vi "Config_Populate.vi"(8 "error in (no error)":errorcluster, 11 "Config Ref In":T1) -> (0 "error out":errorcluster, 3 "refnum out":T1)   [LabVIEW 2021]
uses:
  <vilib>/Utility/config.llb/Config Data RefNum.ctl
  Config_Cluster.ctl
  Mode_Enum.ctl
  <vilib>/Utility/config.llb/Write Key (Path).vi
  <vilib>/Utility/config.llb/Write Key (String).vi
  <vilib>/Utility/config.llb/NI_LVConfig.lvlib
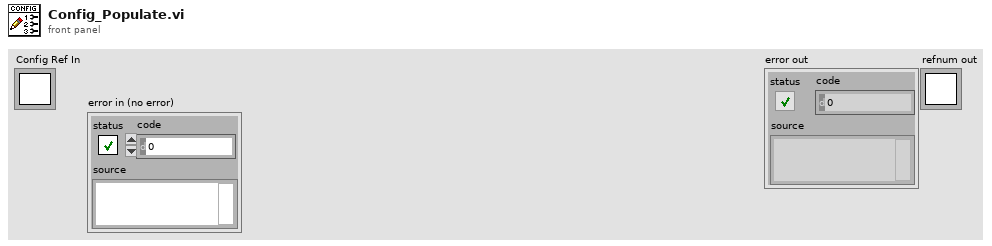
[diagram p1: front panel]
types:
  T1 = typedef "NI_LVConfig.lvlib/Config Data RefNum.ctl" = refnum<k1>
  T2 = typedef "Config_Cluster.ctl" = cluster{"General":cluster{"Config.ini":path, "Default Logging Path":path}, "Hardware":cluster{"Global T VAR":refnum<k21>, "Global B VAR":refnum<k21>, "VISAS":cluster{"GEN COM":refnum<visa-resource-name>, "SCOPE COM":refnum<visa-resource-name>, "VNA COM":refnum<visa-resource-name>}}, "Operation":cluster{"Operation Mode":T3, "Status":string, "NewLog?":bool, "OvenWarn":bool, "Scope Settings":cluster{"TimeBase":dbl, "VerticalScale":dbl}}}
  T3 = typedef "Mode_Enum.ctl" = enum16{"OvenNRDY", "Logging", "Idle-Off", "Idle"}
  T4 = cluster{"Config.ini":path, "Default Logging Path":path}
  T5 = cluster{"Global T VAR":refnum<k21>, "Global B VAR":refnum<k21>, "VISAS":cluster{"GEN COM":refnum<visa-resource-name>, "SCOPE COM":refnum<visa-resource-name>, "VNA COM":refnum<visa-resource-name>}}
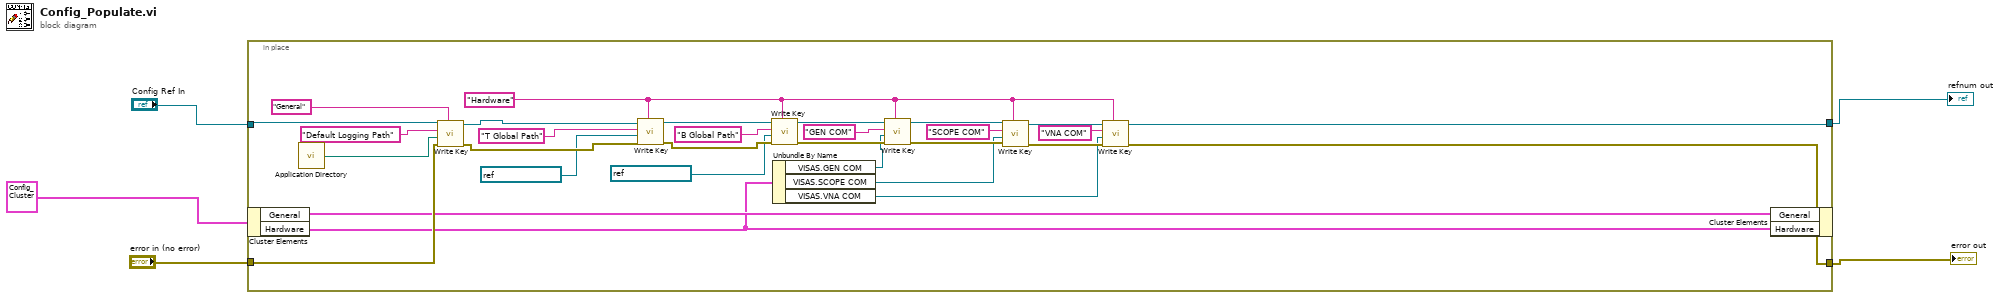
[diagram p0: block diagram]
diagram:
  n1 = in-place {
    in-place-border: "Config Ref In" -> [w35]
    in-place-border: "error in (no error)" -> [w34]
    in-place-border: [w7] -> w2
    in-place-border: [w6] -> w1
    w8 = "Hardware" ("section")
    n2 = in-place-cluster #1(T2 {"General"={"Config.ini"=path "", "Default Logging Path"=path ""}, "Hardware"={"Global T VAR"="", "Global B VAR"="", "VISAS"={"GEN COM"="", "SCOPE COM"="", "VNA COM"=""}}, "Operation"={"Operation Mode"=enum."Logging", "Status"="", "NewLog?"=FALSE, "OvenWarn"=FALSE, "Scope Settings"={"TimeBase"=0.0, "VerticalScale"=4.0}}} ("Configuration Cluster")) -> ("General"=w31:T4, "Hardware"=w12:T5)
    n3 = call <vilib>:"Application Directory.vi"() -> ("Application Directory"=w28:path)
    n4 = call-poly <vilib>:"Write Key.vi"("section"="General", "error in (no error)"=w34, "value"=w28, "key"="Default Logging Path", "refnum"=w35) -> ("error out"=w30:errorcluster, "refnum out"=w32:T1)  [unwired: 4 in, 1 out]
    n5 = call-poly <vilib>:"Write Key.vi"("section"=w8, "error in (no error)"=w30, "value"=refnum<k21> "ni.var.psp://localhost/SV_Temperature/T_VTI_val" ("shared variable refnum in"), "key"="T Global Path", "refnum"=w32) -> ("error out"=w23:errorcluster, "refnum out"=w27:T1)  [unwired: 4 in, 1 out]
    n6 = call-poly <vilib>:"Write Key.vi"("section"=w8, "error in (no error)"=w23, "value"=refnum<k21> "ni.var.psp://localhost/SV_Magnet/B_an_val" ("shared variable refnum in"), "key"="B Global Path", "refnum"=w27) -> ("error out"=w18:errorcluster, "refnum out"=w21:T1)  [unwired: 4 in, 1 out]
    n7 = Unbundle By Name(w12) -> ("VISAS.GEN COM"=w11:refnum<visa-resource-name>, "VISAS.SCOPE COM"=w10:refnum<visa-resource-name>, "VISAS.VNA COM"=w9:refnum<visa-resource-name>)
    n8 = call-poly <vilib>:"Write Key.vi"("section"=w8, "error in (no error)"=w18, "value"=w11, "key"="GEN COM", "refnum"=w21) -> ("error out"=w17:errorcluster, "refnum out"=w20:T1)  [unwired: 4 in, 1 out]
    n9 = call-poly <vilib>:"Write Key.vi"("section"=w8, "error in (no error)"=w17, "value"=w10, "key"="SCOPE COM", "refnum"=w20) -> ("error out"=w16:errorcluster, "refnum out"=w19:T1)  [unwired: 4 in, 1 out]
    n10 = call-poly <vilib>:"Write Key.vi"("section"=w8, "error in (no error)"=w16, "value"=w9, "key"="VNA COM", "refnum"=w19) -> ("error out"=w7:errorcluster, "refnum out"=w6:T1)  [unwired: 4 in, 1 out]
    n11 = in-place-cluster #1("General"=w31, "Hardware"=w12) -> ()  [unwired: 1 out]
  }
  "error out" <- w2
  "refnum out" <- w1
